vi "demo_mrq.vi"   [LabVIEW 2017]
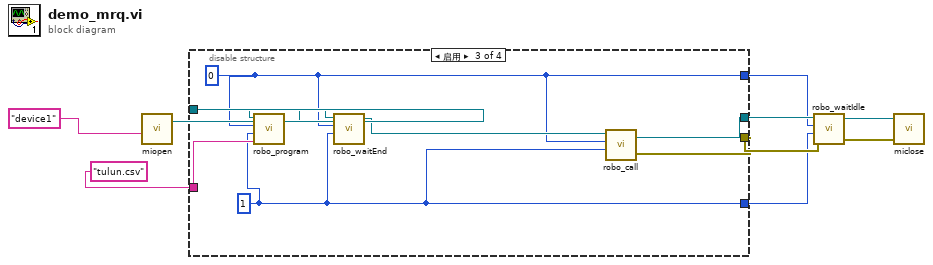
[diagram p0: block diagram]
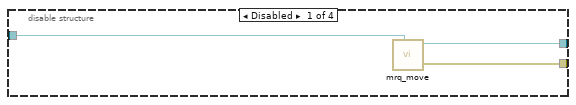
[diagram p2: hidden frame]
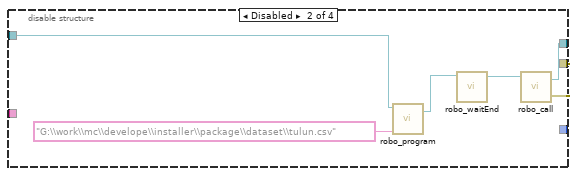
[diagram p3: hidden frame]
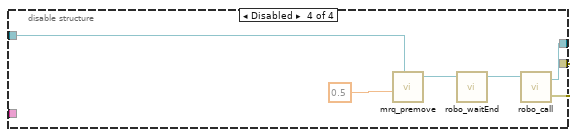
[diagram p4: hidden frame]
diagram:
  n1 = call "miopen.vi"("name"="device1") -> ("VISA资源名称输出"=w8:refnum<visa-resource-name>)  [unwired: 3 in, 1 out]
  n2 = disable-structure shown="启用" {
    disable-tunnel: w8 -> [w12 w15 w24 w32]
    disable-tunnel: [w11 w17 w26 w29] -> w7
    disable-tunnel: [w10 w16 w25 w28] -> w6
    disable-tunnel: "tulun.csv" ("file") -> [_ _ w23 _]
    disable-tunnel: [_ _ w20 _] -> w2
    disable-tunnel: [_ _ w19 _] -> w1
    frame Disabled {
      n3 = call "mrq_move.vi"("VISA资源名称"=w12) -> ("VISA资源名称输出"=w11:refnum<visa-resource-name>, "错误输出"=w10:errorcluster)  [unwired: 6 in]
    }
    frame Disabled {
      n4 = call "robo_program.vi"("VISA资源名称"=w15, "file"="G:\\work\\mc\\develope\\installer\\package\\dataset\\tulun.csv") -> ("VISA资源名称输出"=w14:refnum<visa-resource-name>)  [unwired: 3 in, 1 out]
      n5 = call "robo_waitEnd.vi"("VISA资源名称"=w14) -> ("VISA资源名称输出"=w18:refnum<visa-resource-name>)  [unwired: 4 in, 2 out]
      n6 = call "robo_call.vi"("VISA资源名称"=w18) -> ("错误输出"=w16:errorcluster, "VISA资源名称输出"=w17:refnum<visa-resource-name>)  [unwired: 5 in]
    }
    frame Enabled {
      w19 = 1 ("page")
      w20 = 0 ("ax")
      n7 = call "robo_program.vi"("VISA资源名称"=w24, "ax"=w20, "page"=w19, "file"=w23) -> ("VISA资源名称输出"=w22:refnum<visa-resource-name>)  [unwired: 1 in, 1 out]
      n8 = call "robo_waitEnd.vi"("VISA资源名称"=w22, "ax"=w20, "page"=w19) -> ("VISA资源名称输出"=w21:refnum<visa-resource-name>)  [unwired: 2 in, 2 out]
      n9 = call "robo_call.vi"("page"=w19, "ax"=w20, "VISA资源名称"=w21) -> ("错误输出"=w25:errorcluster, "VISA资源名称输出"=w26:refnum<visa-resource-name>)  [unwired: 3 in]
    }
    frame Disabled {
      n10 = call "mrq_premove.vi"("VISA资源名称"=w32, "t"=sgl 0.5) -> ("VISA资源名称输出"=w31:refnum<visa-resource-name>)  [unwired: 5 in, 1 out]
      n11 = call "robo_waitEnd.vi"("VISA资源名称"=w31) -> ("VISA资源名称输出"=w30:refnum<visa-resource-name>)  [unwired: 4 in, 2 out]
      n12 = call "robo_call.vi"("VISA资源名称"=w30) -> ("错误输出"=w28:errorcluster, "VISA资源名称输出"=w29:refnum<visa-resource-name>)  [unwired: 5 in]
    }
  }
  n13 = call "robo_waitIdle.vi"("VISA资源名称"=w7, "ax"=w2, "page"=w1, "错误输入（无错误）"=w6) -> ("VISA资源名称输出"=w5:refnum<visa-resource-name>, "错误输出"=w4:errorcluster)  [unwired: 1 in, 1 out]
  n14 = call "miclose.vi"("错误输入（无错误）"=w4, "VISA资源名称"=w5) -> ()  [unwired: 1 out]
